vi "PH_Sixpack.Set BaseClass Changes to 6P Configuration.vi"(0 "i ref in":refnum<vi>, 5 "error in":errorcluster) -> (14 "i ref out":refnum<vi>, 16 "Config changed?":bool, 19 "error out":errorcluster)   [LabVIEW 2014, in "PH_Sixpack.lvlib"]
doc: "This VI checks whether base class conditions have been changed which makes it necessary to reconfigure the 6P."
uses:
  PH_Sixpack.lvlib
  PH_Stepmotor_BaseClass/PH_Stepmotor_BaseClass.lvlib
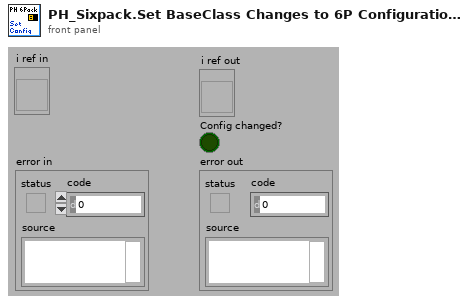
[diagram p1: front panel]
types:
  T1 = typedef "PH_Stepmotor_BaseClass.lvlib/PH_Stepmotor_BaseClass.i attribute.ctl" = cluster{"Device Error":errorcluster, "Axes PSDB Thread":cluster{"Ref":refnum<vi>, "Q-Ref":refnum<queue>, "Data Status":T2}, "Axes":T3[], "Axes PSDB Infos":cluster{"GUI Name":string, "PSDB Instance ID":i32, "PSDB Status Service ID":i32, "Axis":i32, "Class":string}[], "GUI Refs":T8}
  T2 = typedef "PH_PSDBWriter.lvlib/PH_PSDBWriter.Data Status.ctl" = i16
  T3 = typedef "PH_Stepmotor_BaseClass.lvlib/PH_Stepmotor_BaseClass.Axis Attributes.ctl" = cluster{"Settings":T4, "Endswitch?":bool, "DIM Service IDs":T6, "Activity":T7, "Configured?":bool, "Position":cluster{"Current":i32, "Target":i32}, "Position to set":cluster{"New?":bool, "Wanted":i32}, "Stop?":bool, "Reset?":bool, "Move?":bool, "Nothing connected?":bool}
  T4 = typedef "PH_Stepmotor_BaseClass.lvlib/PH_Stepmotor_BaseClass.Axis Settings.ctl" = cluster{"Sign change":bool, "Width":dbl, "Calibration":dbl, "Unit":string, "Motor Type":T5, "Unit Width":string, "Unit CF":string}
  T5 = typedef "PH_Stepmotor_BaseClass.lvlib/PH_Stepmotor_BaseClass.Motor Type.ctl" = enum16{"Unspecific", "OWIS 49.120.2633", "OWIS 49.060.1033", "OWIS 43.040.2558", "Diamond Motion 2200 series", "OWIS 49.120.266B.MV6", "Calorimeter", "Linear Stage 1", "MICOS VT-80", "MICOS VT-80 S", "Standa Rotstage nt0.95A", "PUF RA 320.200", "PUF RA 800.200", "PUF RA 800.400", "PUF RA 400.50", "1324.nn.800.50", "1324.n9c.800.50", "1324.nn.320.200", "1324.nn.400.200", "1324.nn.800.200", "1324.nn.400.50", "1324.8c9c.800.50", "1324.8c9c.400.200"}
  T6 = typedef "PH_Stepmotor_BaseClass.lvlib/PH_Stepmotor_BaseClass.Axis DIM Service IDs.ctl" = cluster{"Settings":i32, "Information":i32}
  T7 = typedef "PH_Stepmotor_BaseClass.lvlib/PH_Stepmotor_BaseClass.Axis Activity.ctl" = enum16{"No Information", "stopped", "running", "Failure", "Alarm", "stopped at backward ES", "stopped at foreward ES"}
  T8 = typedef "PH_Stepmotor_BaseClass.lvlib/PH_Stepmotor_BaseClass.GUI Refs.ctl" = cluster{"Axes Configuration":refnum<vi>, "Device Error":refnum<vi>, "Axes PSDB Infos":refnum<vi>}
  T9 = typedef "Sixpack - Driver.lvlib/Stopswitch Limits.ctl" = cluster{"MinLeft(0)":u16, "MaxRight(1023)":u16}
  T10 = typedef "Sixpack - Driver.lvlib/VmaxAmax.ctl" = cluster{"VMax(511)":u16, "AMax(128)":u16}
  T11 = typedef "Sixpack - Driver.lvlib/Motor Parameter.ctl" = cluster{"Poslimit (6400)":u32, "P5 Bits":T12, "P6 Bits":T13}
  T12 = typedef "Sixpack - Driver.lvlib/MotorParameter_P5.ctl" = cluster{"MT_PI":bool, "MT_ROTARY":bool, "MT_AUTONULLCMD":bool, "MT_TESTNULL":bool, "MT_NULLLEFT":bool, "MT_NULLCENTRE":bool, "MT_STOPNULL":bool, "MT_FILTERSWITCH":bool}
  T13 = typedef "Sixpack - Driver.lvlib/MotorParameter_P6.ctl" = cluster{"MT_OPTIMIZEWAY":bool, "MT_FASTREF":bool, "MT_MECHREF":bool, "MT_DELAYTESTNULL":bool, "MT_STOPSOFT":bool, "MT_STOPNOREF":bool, "MT_NULLPOSITIVE":bool, "MUT_STOPFULSTEPS":bool}
  T14 = typedef "Sixpack - Driver.lvlib/Ref Search Parameter.ctl" = cluster{"VRefMax(100)":u16, "DebouncingTime (22ms)":u8}
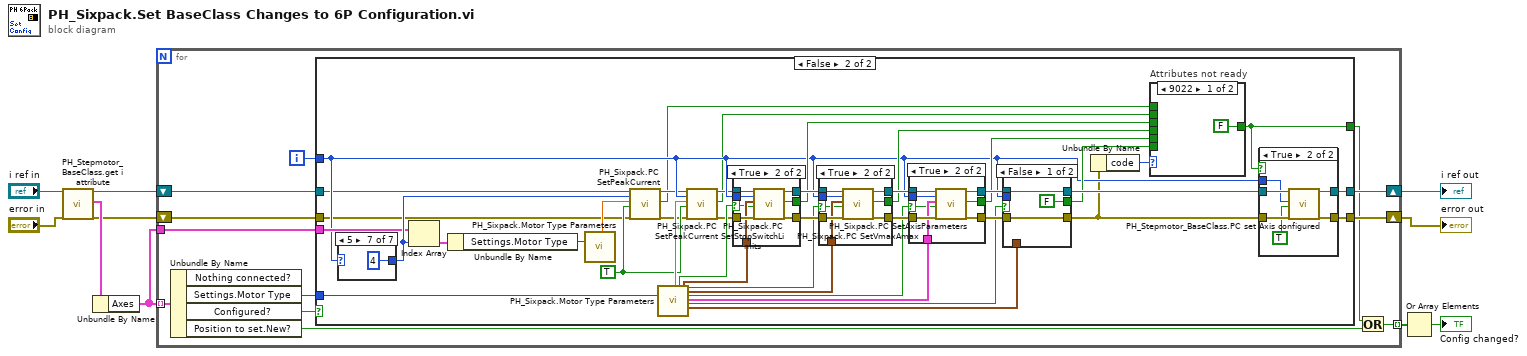
[diagram p0: block diagram]
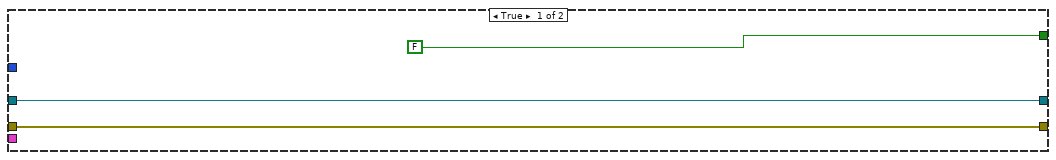
[diagram p2: hidden frame]
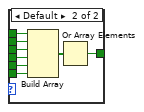
[diagram p3: hidden frame]
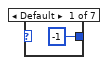
[diagram p4: hidden frame]
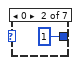
[diagram p5: hidden frame]
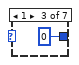
[diagram p6: hidden frame]
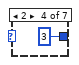
[diagram p7: hidden frame]
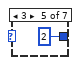
[diagram p8: hidden frame]
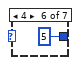
[diagram p9: hidden frame]
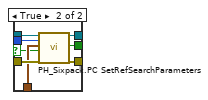
[diagram p11: hidden frame]
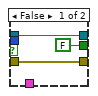
[diagram p12: hidden frame]
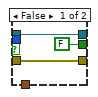
[diagram p13: hidden frame]
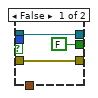
[diagram p14: hidden frame]
diagram:
  n1 = call "PH_Stepmotor_BaseClass.get i attribute.vi"("i ref in"="i ref in", "error in (no error)"="error in") -> ("i ref out"=w2:refnum<vi>, "i attribute"=w8:T1, "error out"=w1:errorcluster)  [unwired: 15 in]
  n2 = Unbundle By Name(w8) -> ("Axes"=w3:T3[])
  n3 = for {
    shift-right: [w18] -> w5
    shift-left: w1 -> [w22]
    shift-right: [w17] -> w6
    shift-left: w2 -> [w19]
    tunnel: w3 -> [w21] mode=indexing
    tunnel: [w15] -> w7 mode=indexing
    tunnel: w3 -> [w11]
    i -> [w16]
    n4 = Unbundle By Name(w21) -> ("Settings.Motor Type"=w20:T5, "Configured?"=w12:bool, "Position to set.New?"=w14:bool)  [unwired: 1 out]
    n5 = case shown="False" w12 {
      tunnel: w22 -> [w24 w30]
      tunnel: w20 -> [_ w57]
      tunnel: w19 -> [w25 w31]
      tunnel: [w24 w52] -> w18
      tunnel: [w25 w50] -> w17
      tunnel: w16 -> [_ w36]
      tunnel: [FALSE w45] -> w13
      tunnel: w11 -> [_ w39]
      frame True {
      }
      frame False {
        w37 = TRUE ("To set?")
        n6 = case shown="5" w36 {
          tunnel: [-1 ("index") 1 ("index") 0 ("index") 3 ("index") 2 ("index") 5 ("index") 4 ("index")] -> w40
          frame Default {
          }
          frame 0 {
          }
          frame 1 {
          }
          frame 2 {
          }
          frame 3 {
          }
          frame 4 {
          }
          frame 5 {
          }
        }
        n7 = Index Array(array=w39, index=w40) -> (element=w43:T3)
        n8 = Unbundle By Name(w43) -> ("Settings.Motor Type"=w42:T5)
        n9 = call "PH_Sixpack.Motor Type Parameters.vi"("Motor Type"=w42) -> ("I max [%]"=w41:dbl)  [unwired: 17 in, 9 out]
        n10 = call "PH_Sixpack.PC SetPeakCurrent.vi"("i ref in"=w31, "Axis"=w40, "Imax (50%)"=w41, "To set?"=w37, "error in"=w30) -> ("i ref out"=w33:refnum<vi>, "ok?"=w28:bool, "error out"=w32:errorcluster)  [unwired: 12 in]
        n11 = call "PH_Sixpack.Motor Type Parameters.vi"("Motor Type"=w57) -> ("I max [%]"=w38:dbl, "Set Stopswitch Limits?"=w44:bool, "Stopswitch Limits"=w60:T9, "Set VmaxAmax"=w56:bool, "VmaxAmax"=w55:T10, "Set Axis Parameter"=w53:bool, "Axis Parameter"=w54:T11, "Set Ref Search Parameters"=w59:bool, "Ref Search Parameters"=w58:T14)  [unwired: 17 in, 1 out]
        n12 = call "PH_Sixpack.PC SetPeakCurrent.vi"("i ref in"=w33, "Axis"=w36, "Imax (50%)"=w38, "To set?"=w37, "error in"=w32) -> ("i ref out"=w35:refnum<vi>, "ok?"=w29:bool, "error out"=w34:errorcluster)  [unwired: 12 in]
        n13 = case shown="True" w44 {
          selector: w44 -> [_ w128]
          tunnel: w35 -> [w125 w134]
          tunnel: w34 -> [w126 w133]
          tunnel: [w125 w132] -> w64
          tunnel: [w126 w131] -> w62
          tunnel: w36 -> [_ w130]
          tunnel: w60 -> [_ w129]
          tunnel: [FALSE ("ok?") w127] -> w49
          frame False {
          }
          frame True {
            n14 = call "PH_Sixpack.PC SetStopSwitchLimits.vi"("i ref in"=w134, "axis"=w130, "Stopswitch Limits"=w129, "To set?"=w128, "error in"=w133) -> ("i ref out"=w132:refnum<vi>, "ok?"=w127:bool, "error out"=w131:errorcluster)  [unwired: 12 in]
          }
        }
        n15 = case shown="True" w56 {
          selector: w56 -> [_ w117]
          tunnel: w64 -> [w115 w123]
          tunnel: [w115 w122] -> w63
          tunnel: w62 -> [w114 w121]
          tunnel: [w114 w120] -> w61
          tunnel: w36 -> [_ w119]
          tunnel: w55 -> [_ w118]
          tunnel: [FALSE ("ok?") w116] -> w48
          frame False {
          }
          frame True {
            n16 = call "PH_Sixpack.PC SetVmaxAmax.vi"("i ref in"=w123, "axis"=w119, "V max A max"=w118, "To Set?"=w117, "error in"=w121) -> ("i ref out"=w122:refnum<vi>, "ok?"=w116:bool, "error out"=w120:errorcluster)  [unwired: 12 in]
          }
        }
        n17 = case shown="True" w53 {
          selector: w53 -> [_ w106]
          tunnel: [w103 w112] -> w66
          tunnel: [w104 w111] -> w65
          tunnel: w63 -> [w104 w110]
          tunnel: w61 -> [w103 w109]
          tunnel: w36 -> [_ w108]
          tunnel: w54 -> [_ w107]
          tunnel: [FALSE ("ok?") w105] -> w47
          frame False {
          }
          frame True {
            n18 = call "PH_Sixpack.PC SetAxisParameters.vi"("i ref in"=w110, "axis"=w108, "Axis Parameter"=w107, "Set?"=w106, "error in (no error)"=w109) -> ("i ref out"=w111:refnum<vi>, "ok?"=w105:bool, "error out"=w112:errorcluster)  [unwired: 12 in]
          }
        }
        n19 = case shown="False" w59 {
          selector: w59 -> [_ w95]
          tunnel: w66 -> [w92 w101]
          tunnel: w65 -> [w93 w100]
          tunnel: [w93 w99] -> w51
          tunnel: [w92 w98] -> w27
          tunnel: w36 -> [_ w97]
          tunnel: w58 -> [_ w96]
          tunnel: [FALSE ("ok?") w94] -> w46
          frame False {
          }
          frame True {
            n20 = call "PH_Sixpack.PC SetRefSearchParameters.vi"("i ref in"=w100, "axis"=w97, "Ref Search Parameter"=w96, "To set?"=w95, "error in"=w101) -> ("i ref out"=w99:refnum<vi>, "ok?"=w94:bool, "error out"=w98:errorcluster)  [unwired: 12 in]
          }
        }
        n21 = Unbundle By Name(w27) -> ("code"=w26:i32)
        n22 = case "Attributes not ready" shown="9022" w26 {
          tunnel: w49 -> [_ w75]
          tunnel: w48 -> [_ w74]
          tunnel: w47 -> [_ w73]
          tunnel: w46 -> [_ w72]
          tunnel: [FALSE w70] -> w45
          tunnel: w29 -> [_ w69]
          tunnel: w28 -> [_ w68]
          frame 9022 {
          }
          frame Default {
            n23 = Build Array(w68, w69, w75, w74, w73, w72) -> (w71:bool[])
            n24 = Or Array Elements(Boolean array=w71) -> (logical OR=w70:bool)
          }
        }
        n25 = case shown="True" w45 {
          tunnel: w27 -> [w83 w90]
          tunnel: [w83 w89] -> w52
          tunnel: w51 -> [w84 w88]
          tunnel: [w84 w87] -> w50
          tunnel: w36 -> [_ w86]
          frame False {
          }
          frame True {
            n26 = call "PH_Stepmotor_BaseClass.PC set Axis configured.vi"("VI in"=w88, "Axis"=w86, "Configured?"=TRUE, "error in (no error)"=w90) -> ("VI out"=w87:refnum<vi>, "error out"=w89:errorcluster)  [unwired: 14 in]
          }
        }
      }
    }
    n27 = Or(x=w13, y=w14) -> (x .or. y?=w15:bool)
  }
  "i ref out" <- w6
  "error out" <- w5
  n28 = Or Array Elements(Boolean array=w7) -> (logical OR=→"Config changed?":bool)
